vi "line_regulation_test.vi"() -> ()   [LabVIEW 2020, in "line_regulation_test.lvlib"]
uses:
  line_regulation_test.lvlib
  typedefs/test_inputs.ctl
  typedefs/test_results.ctl
  typedefs/instrument_resources.ctl
  <vilib>/addons/_JKI Toolkits/State Machine/_JKI_lib_State_Machine.llb/Select State(s)_err__jki_lib_state_machine.vi
  drivers/Agilent 34401/Public/Data/Read (Single Point).vi
  drivers/Agilent 34401/Agilent 34401.lvlib
  drivers/Agilent E364X Series/Agilent E364X Series.lvlib
  drivers/Agilent 3352X Series/Agilent 3352X Series.lvlib
  drivers/Agilent B2900 Series/Agilent B2900 Series.lvlib
panel:
  in  "UI Tab":enum32{"Test", "Instrument Resources"}(tab)
  in  "test_inputs":T1={"Vin 1 (V)"=36.0, "Iin Limit (A)"=0.1, "ILoad (A)"=0.0, "Vdd (V)"=36.0, "IVdd Limit (A)"=0.1, "Vin 2 (V)"=10.0} {"Vin 2 (V)" format="%#_6p"; "IVdd Limit (A)" format="%#_6p"; "Vdd (V)" format="%#_6p"; "ILoad (A)" format="%#_6p"; "Iin Limit (A)" format="%#_6p"; "Vin 1 (V)" format="%#_6p"}
  out "Output Results":T2
  in  "instrument_resources":T3={"Vin Voltage DMM"="Vin_Volt", "Vin Current DMM"="Vin_Current", "Vout Voltage DMM"="Vout Voltage DMM", "Vout Current DMM"="Vout_Current", "Eload"="Eload", "FSW_Source"="FSW", "Vin_supply"="Vin_supply", "Vdd_supply"="Vin_supply"}
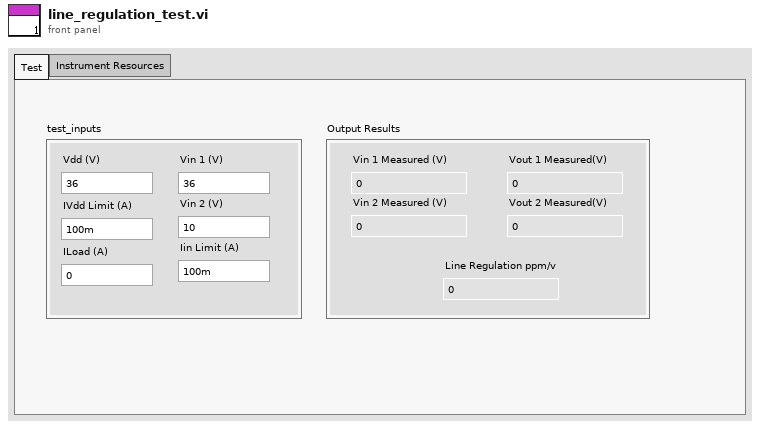
[diagram p1: front panel]
types:
  T1 = typedef "line_regulation_test.lvlib/test_inputs.ctl" = cluster{"Vin 1 (V)":dbl, "Iin Limit (A)":dbl, "ILoad (A)":dbl, "Vdd (V)":dbl, "IVdd Limit (A)":dbl, "Vin 2 (V)":dbl}
  T2 = typedef "line_regulation_test.lvlib/test_results.ctl" = cluster{"Vin 1 Measured (V)":dbl, "Vin 2 Measured (V)":dbl, "Line Regulation ppm/v":dbl, "Vout 1 Measured(V)":dbl, "Vout 2 Measured(V)":dbl}
  T3 = typedef "line_regulation_test.lvlib/instrument_resources.ctl" = cluster{"Vin Voltage DMM":refnum<visa-resource-name>, "Vin Current DMM":refnum<visa-resource-name>, "Vout Voltage DMM":refnum<visa-resource-name>, "Vout Current DMM":refnum<visa-resource-name>, "Eload":refnum<visa-resource-name>, "FSW_Source":refnum<visa-resource-name>, "Vin_supply":refnum<visa-resource-name>, "Vdd_supply":refnum<visa-resource-name>}
  T4 = cluster{"test_inputs":T1, "output_results":T2, "instrument_resources":T3}
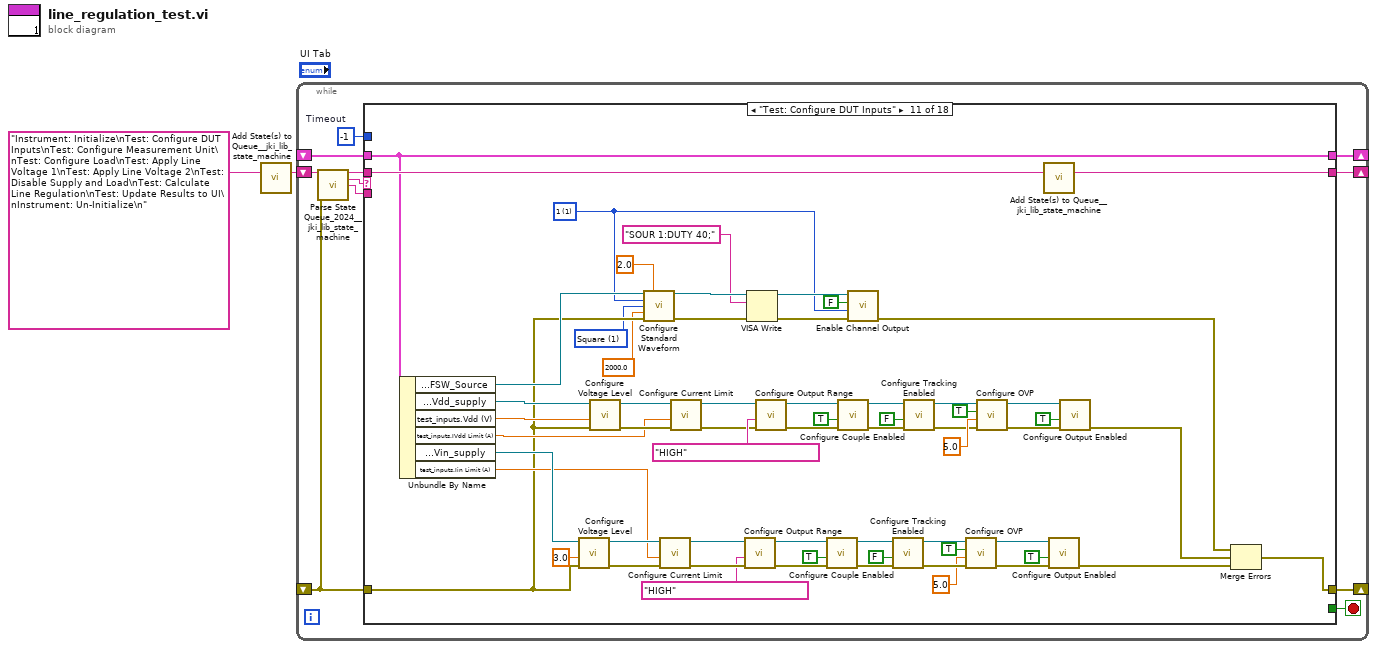
[diagram p0: block diagram]
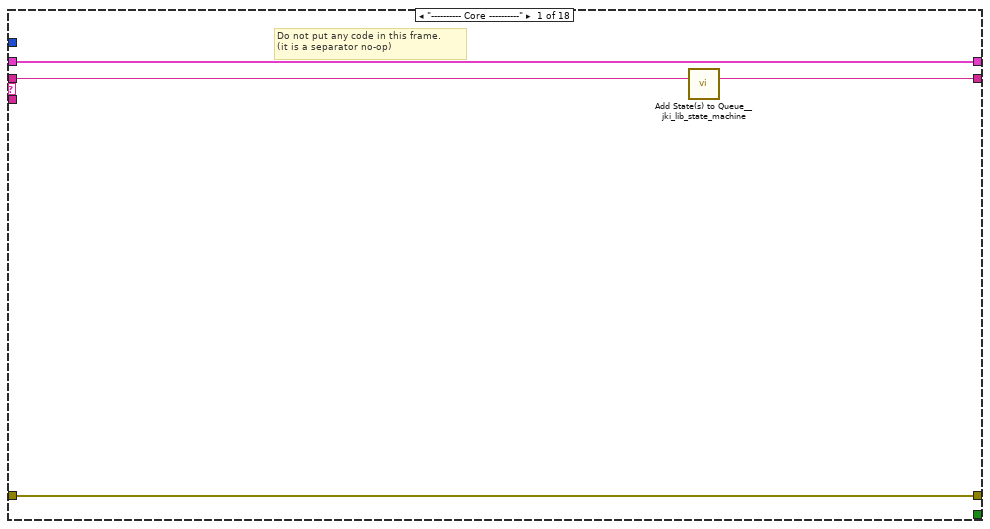
[diagram p2: hidden frame]
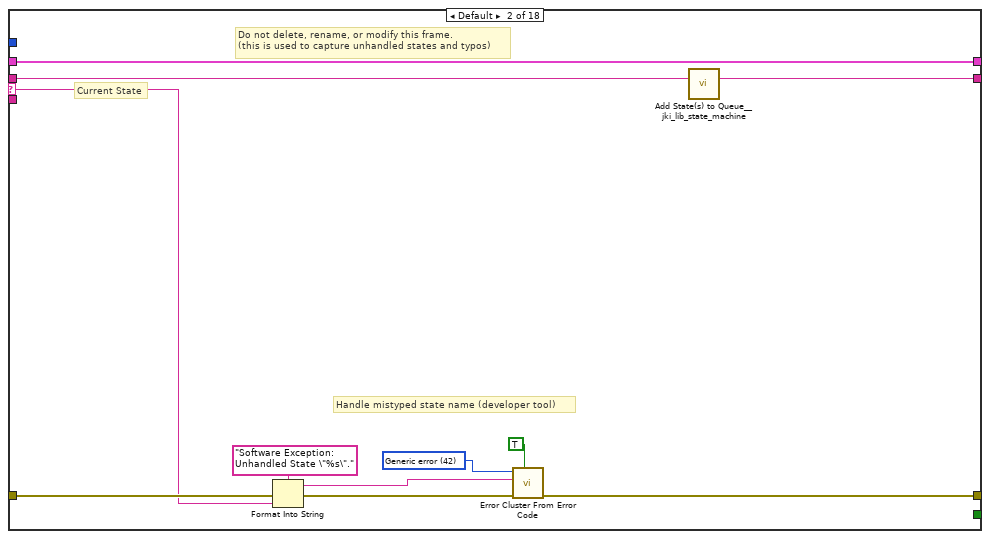
[diagram p3: hidden frame]
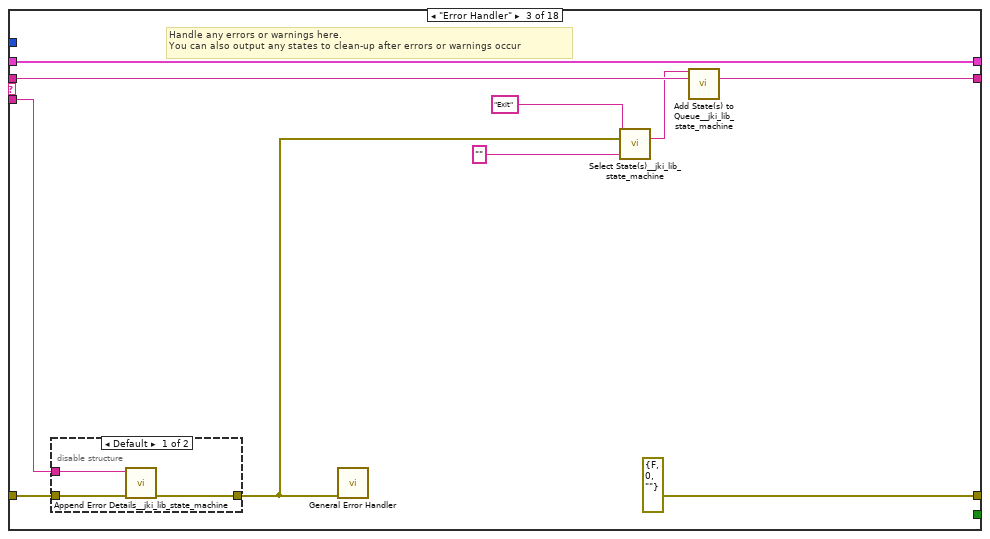
[diagram p4: hidden frame]
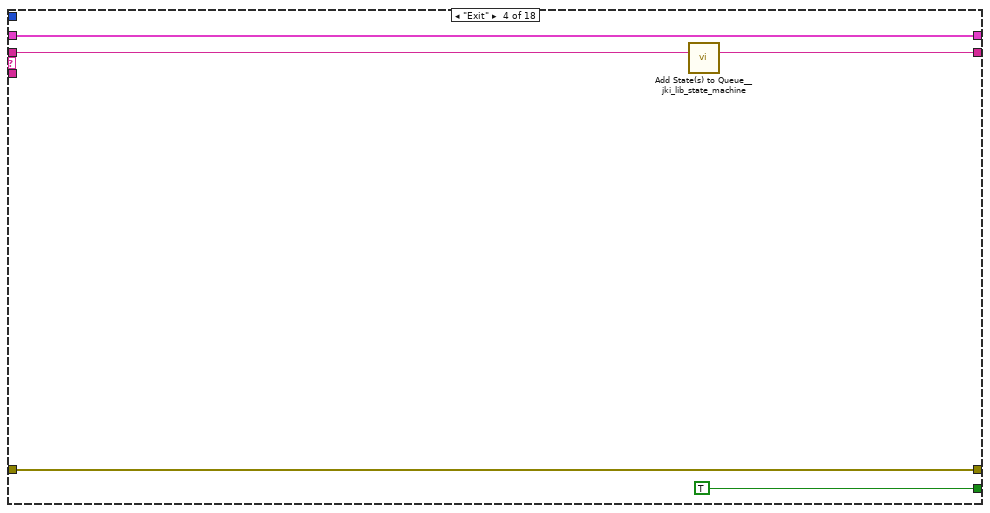
[diagram p6: hidden frame]
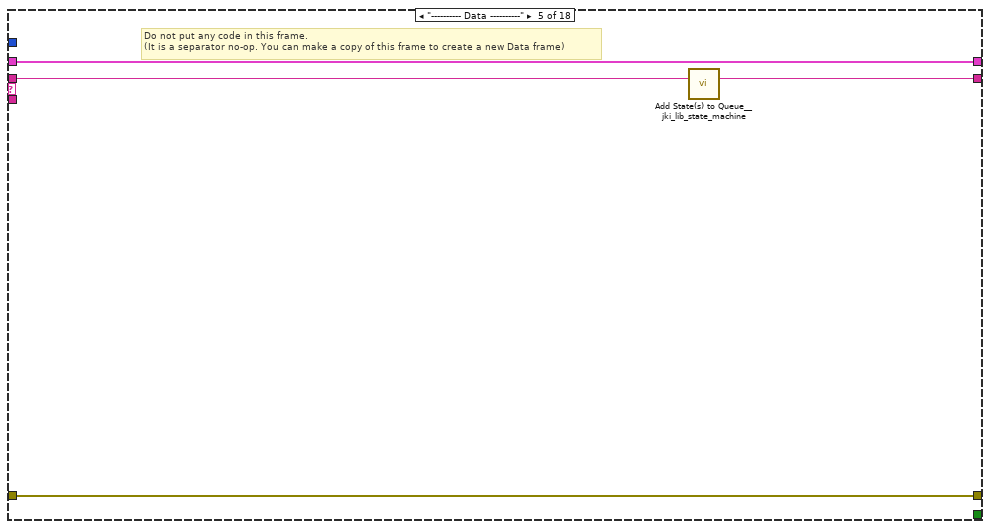
[diagram p7: hidden frame]
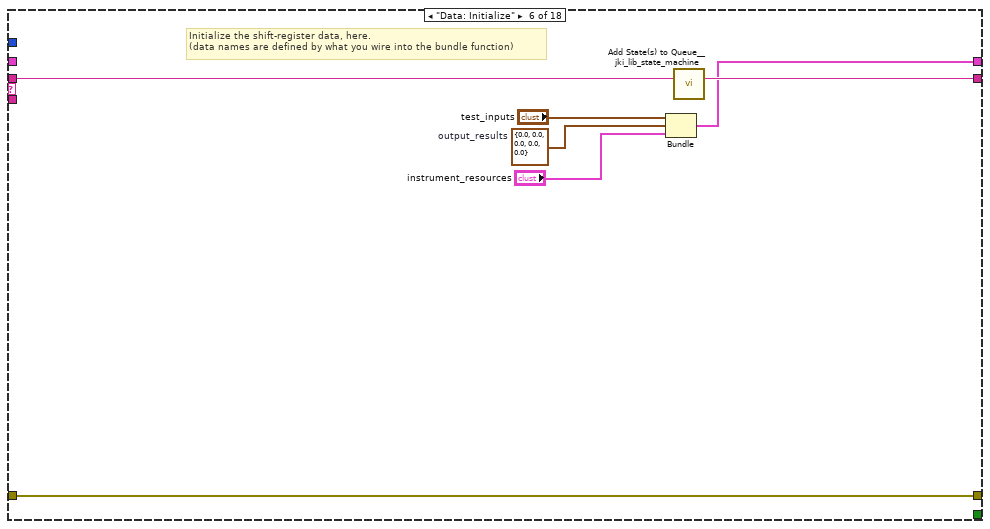
[diagram p8: hidden frame]
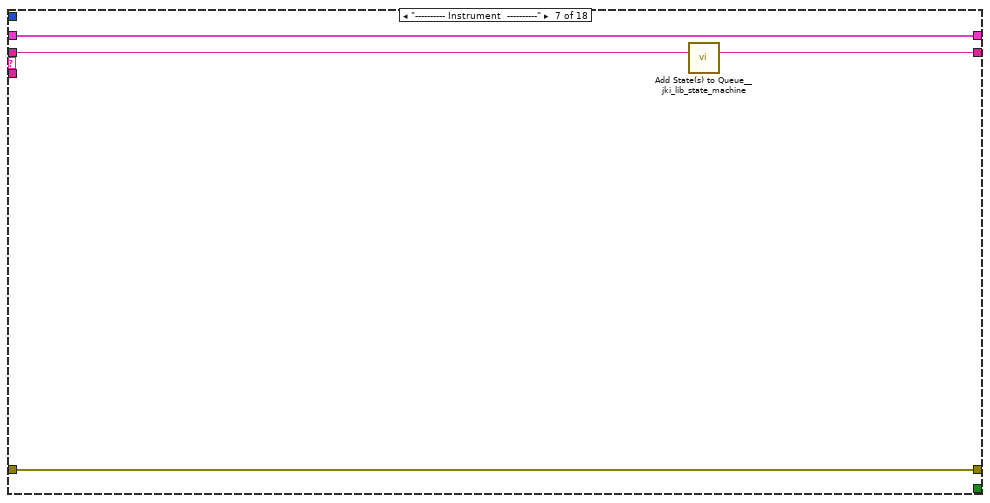
[diagram p9: hidden frame]
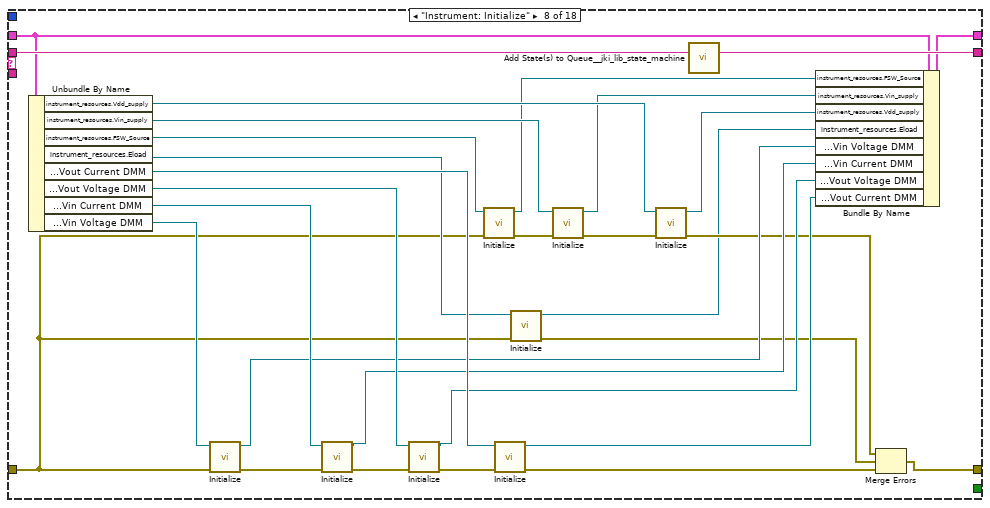
[diagram p10: hidden frame]
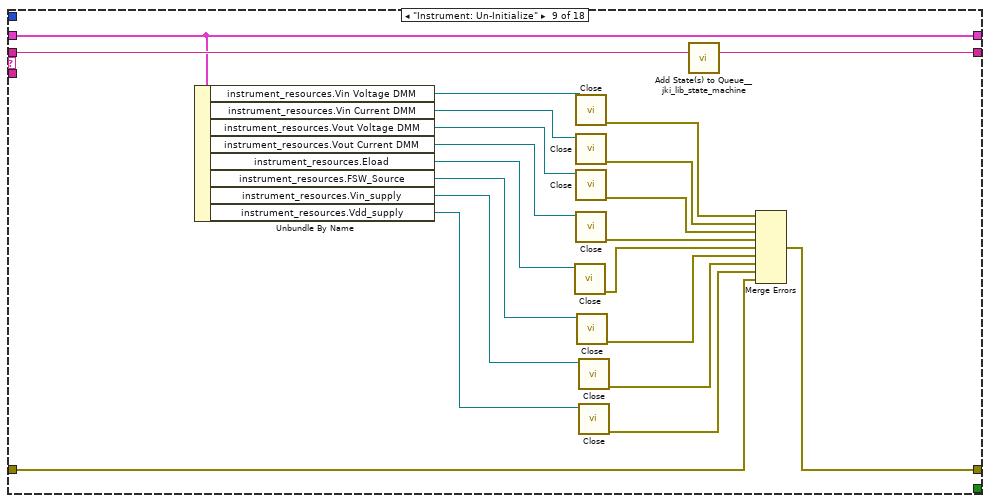
[diagram p11: hidden frame]
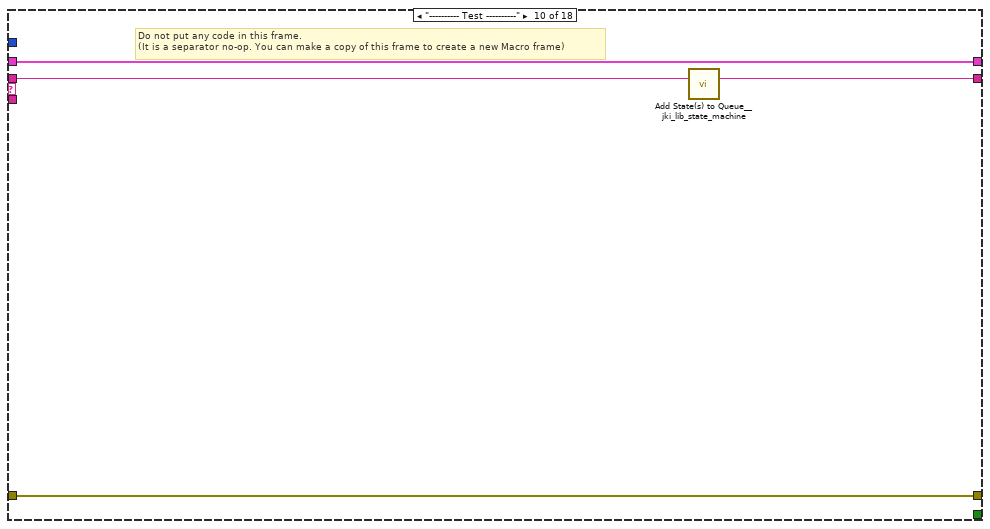
[diagram p12: hidden frame]
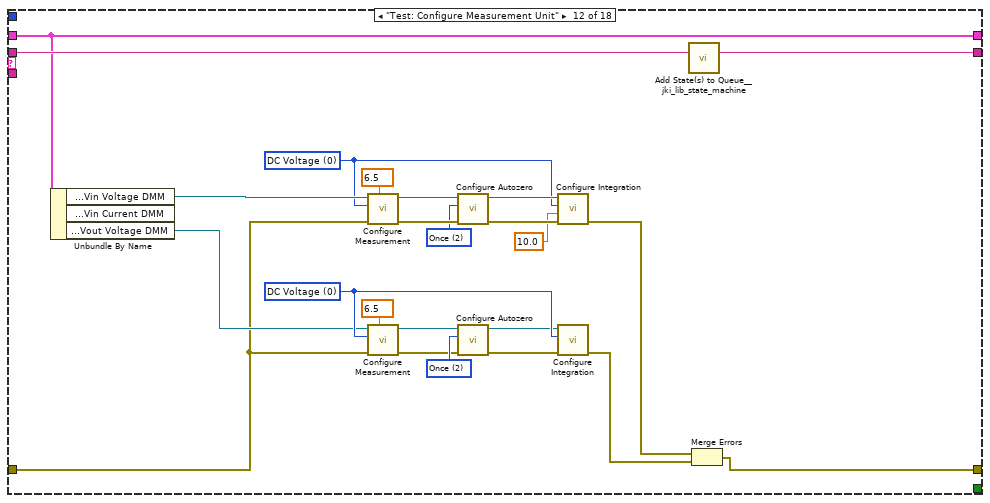
[diagram p13: hidden frame]
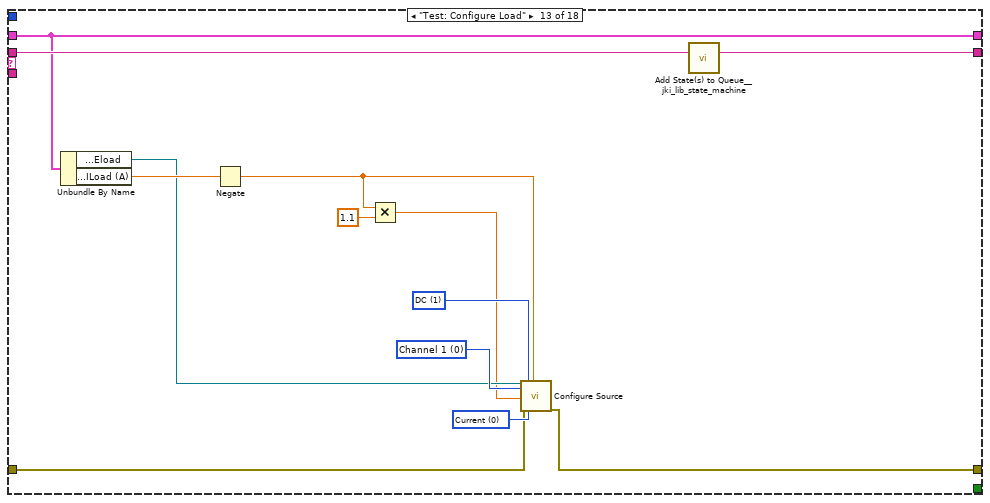
[diagram p14: hidden frame]
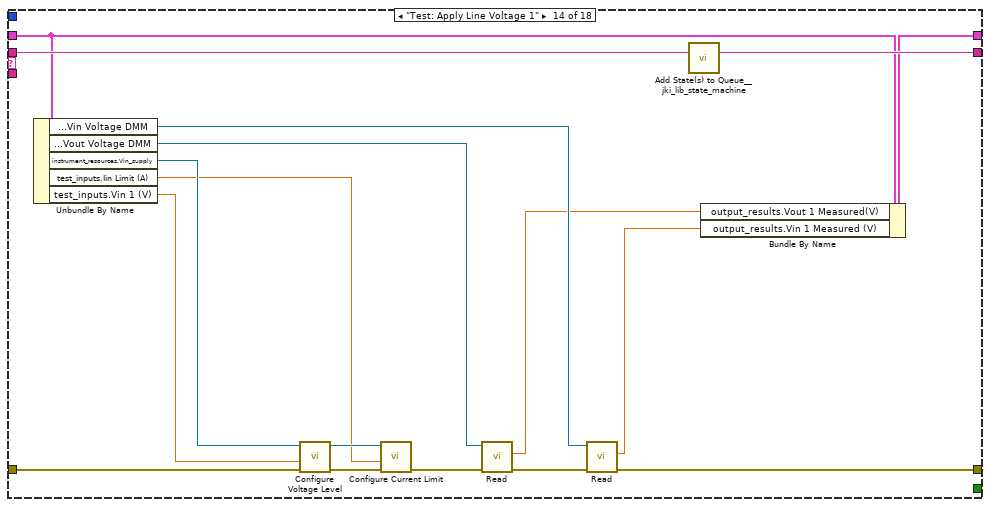
[diagram p15: hidden frame]
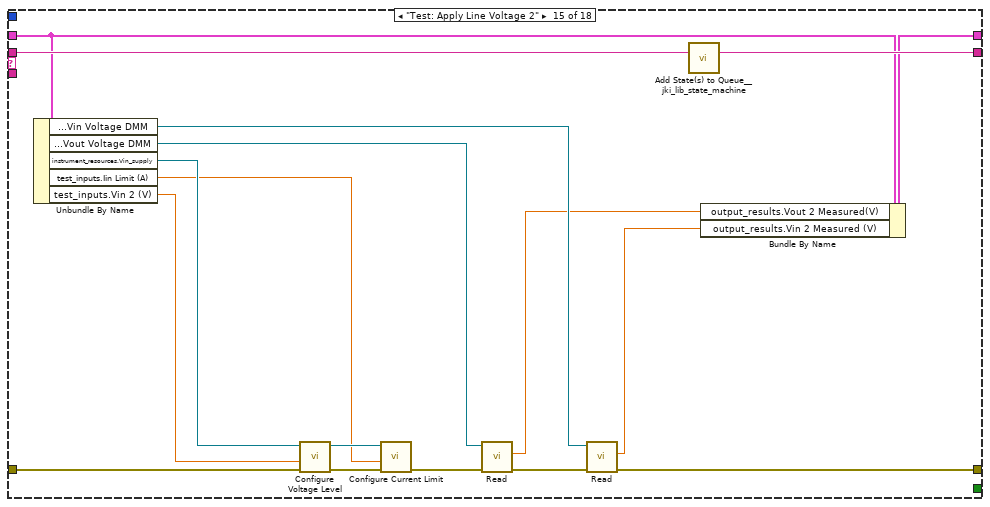
[diagram p16: hidden frame]
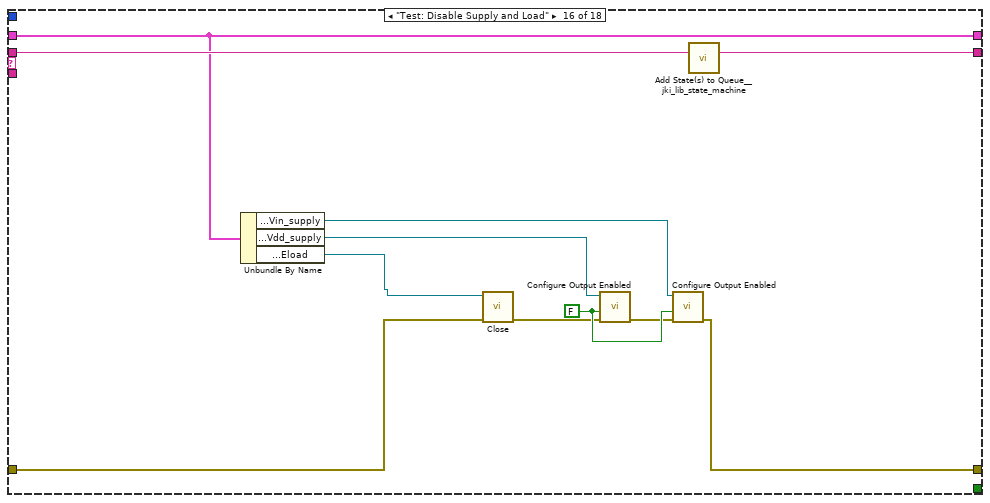
[diagram p17: hidden frame]
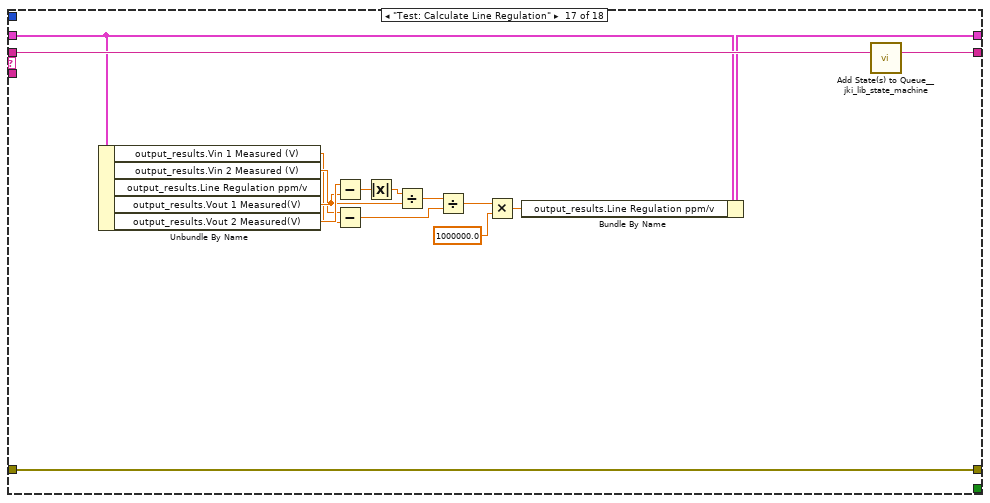
[diagram p18: hidden frame]
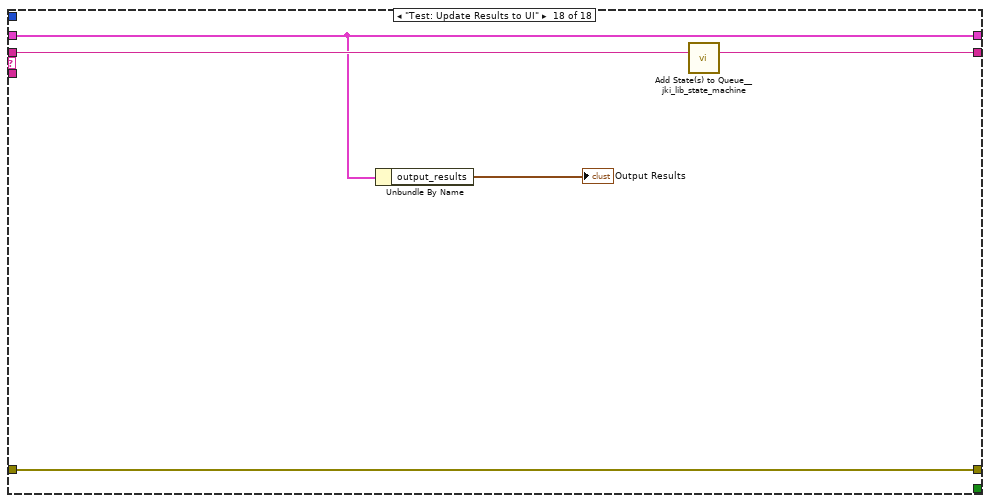
[diagram p19: hidden frame]
diagram:
  n1 = call <vilib>:"Add State(s) to Queue__jki_lib_state_machine.vi"("State(s) in (\"\")"="Instrument: Initialize\nTest: Configure DUT Inputs\nTest: Configure Measurement Unit\nTest: Configure Load\nTest: Apply Line Voltage 1\nTest: Apply Line Voltage 2\nTest: Disable Supply and Load\nTest: Calculate Line Regulation\nTest: Update Results to UI\nInstrument: Un-Initialize\n") -> ("States Out"=w2:string)  [unwired: 14 in]
  n2 = while {
    shift-right: [w6] -> _
    shift-left: _ -> [w5]
    shift-right: [w9] -> _
    shift-left: _ -> [w3]
    shift-right: [w8] -> _
    shift-left: w2 -> [w10]
    stop <- w7 stop-if-true
    w4 = -1  # Timeout
    n3 = call <vilib>:"Parse State Queue_2024__jki_lib_state_machine.vi"("State Queue"=w10, "Error In (no error)"=w3) -> ("Remaining States"=w12:string, "Current State"=w13:string, "Arguments"=w11:string)  [unwired: 11 in]
    n4 = case shown="\"Test: Configure DUT Inputs\"" w13 {
      selector: w13 -> [_ w18 _ _ _ _ _ _ _ _ _ _ _ _ _ _ _ _]
      tunnel: w12 -> [w17 w22 w38 w47 w51 w58 w62 w92 w113 w117 w178 w202 w215 w232 w249 w260 w276 w281]
      tunnel: w11 -> [_ _ w33 _ _ _ _ _ _ _ _ _ _ _ _ _ _ _]
      tunnel: w5 -> [w14 w20 w35 w45 w48 _ w59 w70 w111 w114 w176 w200 w213 w219 w236 w258 w272 w278]
      tunnel: [w15 w24 errorcluster {"status"=FALSE, "code"=0, "source"=""} ("error out") w44 w49 w55 w60 w67 w96 w115 w124 w180 w206 w217 w234 w253 w274 w279] -> w9
      tunnel: w3 -> [w15 w23 w34 w44 w49 w55 w60 w64 w95 w115 w133 w182 w207 w228 w245 w252 w274 w279]
      tunnel: [w16 w21 w37 w46 w50 w57 w61 w91 w112 w116 w177 w201 w214 w231 w248 w259 w275 w280] -> w8
      tunnel: [_ _ _ TRUE _ _ _ _ _ _ _ _ _ _ _ _ _ _] -> w7
      tunnel: [w14 w20 w35 w45 w48 w56 w59 w71 w111 w114 w176 w200 w213 w220 w237 w258 w273 w278] -> w6
      tunnel: w4 -> [_ _ _ _ _ _ _ _ _ _ _ _ _ _ _ _ _ _]
      frame "---------- Core ----------" {
        # "Do not put any code in this frame.\n(it is a separator no-op)"
        n5 = call <vilib>:"Add State(s) to Queue__jki_lib_state_machine.vi"("State(s) in (\"\")"=w17) -> ("States Out"=w16:string)  [unwired: 14 in]
      }
      frame Default {
        w27 = 42 items=["No error", "Argument error", "Memory is full", "Out of zone", "End of file", "File already open", "Generic file I/O error", "File not found", "File permission error", "Disk is full", "Duplicate path", "Too many files open", "System feature not enabled", "Resource file not found", "Cannot add resource", "Resource not found", "Image not found", "Image memory error", "Pen does not exist", "Config type invalid", "Config token not found", "Config parse error", "Config memory error", "Bad external code format", "Bad external code offset", "External code not present", "Null window", "Destroy window error", "Null menu", "Print aborted", "Bad print record", "Print driver error", "Windows error during printing", "Memory error during printing", "Print dialog error", "Generic print error", "Invalid device refnum", "Device not found", "Device parameter error", "Device unit error", "Cannot open device", "Device call aborted", "Generic error", "Cancelled by user", "Object ID too low", "Object ID too high", "Object not in heap", "Unknown heap", "Unknown object (invalid DefProc)", "Unknown object (DefProc not in table)", "Message out of range", "Invalid (null) method", "Unknown message", "Manager call not supported", "Bad address", "Network operation in progress", "Network operation timed out", "Connection is busy", "Network attribute not supported", "Network error", "Address in use", "System out of memory", "Connection aborted", "Connection refused", "Not connected", "Already connected", "Connection closed", "Initialization error (interapplication manager)", "Bad occurrence", "Wait on unbound occurrence handler", "Occurrence queue overflow", "Datalog type conflict", "Unused", "Unrecognized type (interapplication manager)", "Memory corrupt", "Failed to make temporary DLL", "Old CIN version", "Drag socket not found", "Failed to load drop-object", "Failed to register OLE object", "Failed to release OLE object", "Format specifier type mismatch", "Unknown format specifier", "Too few format specifiers", "Too many format specifiers", "Scan failed", "Newer CIN version", "Error converting to variant", "Runtime menu error", "Password tampered", "Variant attribute not found", "Incompatible variant data type", "Event data is not available", "Event Store is not present", "Occurrence is not found", "Event Queue is not created", "Event info is not available", "Refnum passed is NULL", "Error retrieving Class GUID", "Error retrieving CoClass GUID", "Error retrieving TypeLib GUID.", "Bad built application magic bytes.", "Specific driver is different from the specific driver associated with the Logical Name.", "There is no session opened to the class driver.", "Max Error", "MAX - Error with config objects", "MAX - Error loading configuration", "MAX - Group not supported"]
        # "Current State"
        # "Do not delete, rename, or modify this frame.\n(this is used to capture unhandled states and typos)"
        # "Handle mistyped state name (developer tool)"
        n6 = Format Into String(format string="Software Exception: Unhandled State \"%s\"." ("message"), error in=w23, w18) -> (resulting string=w26:string, error out=w25:errorcluster)  [unwired: 1 in]
        n7 = call <vilib>:"Error Cluster From Error Code.vi"("show call chain? (False)"=TRUE, "error in (no error)"=w25, "error message (\"\")"=w26, "error code (0)"=w27) -> ("error out"=w24:errorcluster)  [unwired: 5 in]
        n8 = call <vilib>:"Add State(s) to Queue__jki_lib_state_machine.vi"("State(s) in (\"\")"=w22) -> ("States Out"=w21:string)  [unwired: 14 in]
      }
      frame "Error Handler" {
        # "Handle any errors or warnings here.\nYou can also output any states to clean-up after errors or warnings occur"
        n9 = disable-structure shown="Default" {
          disable-tunnel: w34 -> [w41 w42]
          disable-tunnel: w33 -> [w40 _]
          disable-tunnel: [w39 w42] -> w32
          frame condition #0 (active) {
            n10 = call <vilib>:"Append Error Details__jki_lib_state_machine.vi"("error in (no error)"=w41, "Previous State and Argument(s)"=w40) -> ("error out"=w39:errorcluster)  [unwired: 9 in]
          }
          frame condition #1 {
          }
        }
        n11 = call <vilib>:"General Error Handler.vi"("error in (no error)"=w32) -> ()  [unwired: 10 in, 5 out]
        n12 = call-poly <vilib>:"Select State(s)__jki_lib_state_machine.vi"("State(s) if True (\"\")"="Exit", "Select"=w32, "State(s) if False (\"\")"="") -> ("States Out"=w30:string)  [unwired: 12 in]
        n13 = call <vilib>:"Add State(s) to Queue__jki_lib_state_machine.vi"("State(s) in Front (\"\")"=w30, "State(s) in (\"\")"=w38) -> ("States Out"=w37:string)  [unwired: 13 in]
      }
      frame "Exit" {
        n14 = call <vilib>:"Add State(s) to Queue__jki_lib_state_machine.vi"("State(s) in (\"\")"=w47) -> ("States Out"=w46:string)  [unwired: 14 in]
      }
      frame "---------- Data ----------" {
        # "Do not put any code in this frame.\n(It is a separator no-op. You can make a copy of this frame to create a new Data frame)"
        n15 = call <vilib>:"Add State(s) to Queue__jki_lib_state_machine.vi"("State(s) in (\"\")"=w51) -> ("States Out"=w50:string)  [unwired: 14 in]
      }
      frame "Data: Initialize" {
        w53 = T2 {"Vin 1 Measured (V)"=0.0, "Vin 2 Measured (V)"=0.0, "Line Regulation ppm/v"=0.0, "Vout 1 Measured(V)"=0.0, "Vout 2 Measured(V)"=0.0}  # output_results
        # "Initialize the shift-register data, here.\n(data names are defined by what you wire into the bundle function)"
        n16 = Bundle("test_inputs"="test_inputs", "output_results"=w53, "instrument_resources"="instrument_resources") -> (w56:T4)  [unwired: 1 in]
        n17 = call <vilib>:"Add State(s) to Queue__jki_lib_state_machine.vi"("State(s) in (\"\")"=w58) -> ("States Out"=w57:string)  [unwired: 14 in]
      }
      frame "---------- Instrument  ----------" {
        n18 = call <vilib>:"Add State(s) to Queue__jki_lib_state_machine.vi"("State(s) in (\"\")"=w62) -> ("States Out"=w61:string)  [unwired: 14 in]
      }
      frame "Instrument: Initialize" {
        n19 = Unbundle By Name(w70) -> ("instrument_resources.Vdd_supply"=w83:refnum<visa-resource-name>, "instrument_resources.Vin_supply"=w84:refnum<visa-resource-name>, "instrument_resources.FSW_Source"=w85:refnum<visa-resource-name>, "instrument_resources.Eload"=w66:refnum<visa-resource-name>, "instrument_resources.Vout Current DMM"=w79:refnum<visa-resource-name>, "instrument_resources.Vout Voltage DMM"=w80:refnum<visa-resource-name>, "instrument_resources.Vin Current DMM"=w81:refnum<visa-resource-name>, "instrument_resources.Vin Voltage DMM"=w82:refnum<visa-resource-name>)
        n20 = call "Initialize.vi"("error in (no error)"=w64, "VISA resource name"=w82) -> ("error out"=w88:errorcluster, "VISA resource name out"=w75:refnum<visa-resource-name>)  [unwired: 8 in]
        n21 = call "Initialize.vi"("error in (no error)"=w88, "VISA resource name"=w81) -> ("error out"=w90:errorcluster, "VISA resource name out"=w74:refnum<visa-resource-name>)  [unwired: 8 in]
        n22 = call "Initialize.vi"("error in (no error)"=w90, "VISA resource name"=w80) -> ("error out"=w89:errorcluster, "VISA resource name out"=w73:refnum<visa-resource-name>)  [unwired: 8 in]
        n23 = call "Initialize.vi"("error in (no error)"=w64, "VISA resource name"=w85) -> ("error out"=w87:errorcluster, "VISA resource name out"=w78:refnum<visa-resource-name>)  [unwired: 8 in]
        n24 = call "Initialize.vi"("error in (no error)"=w89, "VISA resource name"=w79) -> ("error out"=w68:errorcluster, "VISA resource name out"=w72:refnum<visa-resource-name>)  [unwired: 8 in]
        n25 = call "Initialize.vi"("error in (no error)"=w64, "VISA resource name"=w66) -> ("error out"=w63:errorcluster, "VISA resource name out"=w65:refnum<visa-resource-name>)  [unwired: 8 in]
        n26 = call "Initialize.vi"("error in (no error)"=w87, "VISA resource name"=w84) -> ("error out"=w86:errorcluster, "VISA resource name out"=w77:refnum<visa-resource-name>)  [unwired: 8 in]
        n27 = call "Initialize.vi"("error in (no error)"=w86, "VISA resource name"=w83) -> ("error out"=w69:errorcluster, "VISA resource name out"=w76:refnum<visa-resource-name>)  [unwired: 8 in]
        n28 = call <vilib>:"Add State(s) to Queue__jki_lib_state_machine.vi"("State(s) in (\"\")"=w92) -> ("States Out"=w91:string)  [unwired: 14 in]
        n29 = Bundle By Name(cluster=w70, "instrument_resources.FSW_Source"=w78, "instrument_resources.Vin_supply"=w77, "instrument_resources.Vdd_supply"=w76, "instrument_resources.Eload"=w65, "instrument_resources.Vin Voltage DMM"=w75, "instrument_resources.Vin Current DMM"=w74, "instrument_resources.Vout Voltage DMM"=w73, "instrument_resources.Vout Current DMM"=w72) -> (w71:T4)
        n30 = Merge Errors(w69, w63, w68) -> (w67:errorcluster)
      }
      frame "Instrument: Un-Initialize" {
        n31 = Unbundle By Name(w111) -> ("instrument_resources.Vin Voltage DMM"=w110:refnum<visa-resource-name>, "instrument_resources.Vin Current DMM"=w109:refnum<visa-resource-name>, "instrument_resources.Vout Voltage DMM"=w108:refnum<visa-resource-name>, "instrument_resources.Vout Current DMM"=w107:refnum<visa-resource-name>, "instrument_resources.Eload"=w94:refnum<visa-resource-name>, "instrument_resources.FSW_Source"=w106:refnum<visa-resource-name>, "instrument_resources.Vin_supply"=w105:refnum<visa-resource-name>, "instrument_resources.Vdd_supply"=w104:refnum<visa-resource-name>)
        n32 = call "Close.vi"("VISA resource name"=w94) -> ("error out"=w93:errorcluster)  [unwired: 10 in]
        n33 = call "Close.vi"("VISA resource name"=w110) -> ("error out"=w103:errorcluster)  [unwired: 10 in]
        n34 = call "Close.vi"("VISA resource name"=w109) -> ("error out"=w102:errorcluster)  [unwired: 10 in]
        n35 = call "Close.vi"("VISA resource name"=w108) -> ("error out"=w101:errorcluster)  [unwired: 10 in]
        n36 = call "Close.vi"("VISA resource name"=w107) -> ("error out"=w100:errorcluster)  [unwired: 10 in]
        n37 = call "Close.vi"("VISA resource name"=w106) -> ("error out"=w99:errorcluster)  [unwired: 10 in]
        n38 = call "Close.vi"("VISA resource name"=w105) -> ("error out"=w98:errorcluster)  [unwired: 10 in]
        n39 = call "Close.vi"("VISA resource name"=w104) -> ("error out"=w97:errorcluster)  [unwired: 10 in]
        n40 = call <vilib>:"Add State(s) to Queue__jki_lib_state_machine.vi"("State(s) in (\"\")"=w113) -> ("States Out"=w112:string)  [unwired: 14 in]
        n41 = Merge Errors(w103, w102, w101, w100, w93, w99, w98, w97, w95) -> (w96:errorcluster)
      }
      frame "---------- Test ----------" {
        # "Do not put any code in this frame.\n(It is a separator no-op. You can make a copy of this frame to create a new Macro frame)"
        n42 = call <vilib>:"Add State(s) to Queue__jki_lib_state_machine.vi"("State(s) in (\"\")"=w117) -> ("States Out"=w116:string)  [unwired: 14 in]
      }
      frame "Test: Configure DUT Inputs" {
        w122 = 1 items=["Sine"=0, "Square"=1, "Ramp"=2, "Noise"=3, "DC"=4, "Triangle"=5, "Pulse"=6, "Sinc"=11, "D-Lorentz"=12, "Gaussian"=13, "Expo Fall"=14, "Expo Rise"=15, "Haversine"=16] ("Waveform Function (0: Sine)")
        w120 = 1 items=["1"=1, "2"=2] ("Channel (1: 1)")
        n43 = Unbundle By Name(w176) -> ("instrument_resources.FSW_Source"=w134:refnum<visa-resource-name>, "instrument_resources.Vdd_supply"=w137:refnum<visa-resource-name>, "test_inputs.Vdd (V)"=w136:dbl, "test_inputs.IVdd Limit (A)"=w135:dbl, "instrument_resources.Vin_supply"=w175:refnum<visa-resource-name>, "test_inputs.Iin Limit (A)"=w156:dbl)
        n44 = call "Configure Voltage Level.vi"("error in (no error)"=w133, "Level (0.0 Volts)"=3.0, "VISA resource name"=w175) -> ("error out"=w174:errorcluster, "VISA resource name out"=w170:refnum<visa-resource-name>)  [unwired: 7 in]
        n45 = call "Configure Voltage Level.vi"("error in (no error)"=w133, "Level (0.0 Volts)"=w136, "VISA resource name"=w137) -> ("error out"=w138:errorcluster, "VISA resource name out"=w142:refnum<visa-resource-name>)  [unwired: 7 in]
        n46 = call "Configure Standard Waveform.vi"("VISA resource name"=w134, "Amplitude (0.1 Vpp)"=2.0, "Channel (1: 1)"=w120, "Waveform Function (0: Sine)"=w122, "Frequency/Sample Rate/Bandwidth (1000 Hz)"=2000.0, "error in (no error)"=w133) -> ("VISA resource name out"=w130:refnum<visa-resource-name>, "error out"=w132:errorcluster)  [unwired: 8 in]
        n47 = call "Configure Current Limit.vi"("error in (no error)"=w174, "Current Limit (0.0 Amps)"=w156, "VISA resource name"=w170) -> ("error out"=w173:errorcluster, "VISA resource name out"=w169:refnum<visa-resource-name>)  [unwired: 7 in]
        n48 = call "Configure Current Limit.vi"("error in (no error)"=w138, "Current Limit (0.0 Amps)"=w135, "VISA resource name"=w142) -> ("error out"=w139:errorcluster, "VISA resource name out"=w143:refnum<visa-resource-name>)  [unwired: 7 in]
        n49 = call "Configure Output Range.vi"("error in (no error)"=w173, "Range (High Voltage / Low Current)"="HIGH", "VISA resource name"=w169) -> ("error out"=w172:errorcluster, "VISA resource name out"=w168:refnum<visa-resource-name>)  [unwired: 7 in]
        n50 = VISA Write(VISA resource name=w130, write buffer="SOUR 1:DUTY 40;", error in (no error)=w132) -> (VISA resource name out=w129:refnum<visa-resource-name>, error out=w131:errorcluster)  [unwired: 1 out]
        n51 = call "Configure Output Range.vi"("error in (no error)"=w139, "Range (High Voltage / Low Current)"="HIGH", "VISA resource name"=w143) -> ("error out"=w140:errorcluster, "VISA resource name out"=w144:refnum<visa-resource-name>)  [unwired: 7 in]
        n52 = call "Configure Couple Enabled.vi"("error in (no error)"=w172, "Coupling Enabled (F: Off)"=TRUE, "VISA resource name"=w168) -> ("error out"=w171:errorcluster, "VISA resource name out"=w167:refnum<visa-resource-name>)  [unwired: 7 in]
        n53 = call "Configure Couple Enabled.vi"("error in (no error)"=w140, "Coupling Enabled (F: Off)"=TRUE, "VISA resource name"=w144) -> ("error out"=w141:errorcluster, "VISA resource name out"=w145:refnum<visa-resource-name>)  [unwired: 7 in]
        n54 = call "Enable Channel Output.vi"("error in (no error)"=w131, "Channel (1: 1)"=w120, "Enable Output (T: Enable)"=FALSE ("Enable Output  (T: Enable)"), "VISA resource name"=w129) -> ("error out"=w125:errorcluster)  [unwired: 6 in, 1 out]
        n55 = call "Configure Tracking Enabled.vi"("error in (no error)"=w171, "Tracking Enabled (F: Off)"=FALSE, "VISA resource name"=w167) -> ("error out"=w163:errorcluster, "VISA resource name out"=w161:refnum<visa-resource-name>)  [unwired: 7 in]
        n56 = call "Configure Tracking Enabled.vi"("error in (no error)"=w141, "Tracking Enabled (F: Off)"=FALSE, "VISA resource name"=w145) -> ("error out"=w149:errorcluster, "VISA resource name out"=w151:refnum<visa-resource-name>)  [unwired: 7 in]
        n57 = call "Configure OVP.vi"("error in (no error)"=w163, "Limit (22.0 Volts)"=5.0, "OVP Enabled (T: On)"=TRUE, "VISA resource name"=w161) -> ("error out"=w159:errorcluster, "VISA resource name out"=w158:refnum<visa-resource-name>)  [unwired: 6 in]
        n58 = call "Configure OVP.vi"("error in (no error)"=w149, "Limit (22.0 Volts)"=5.0, "OVP Enabled (T: On)"=TRUE, "VISA resource name"=w151) -> ("error out"=w153:errorcluster, "VISA resource name out"=w154:refnum<visa-resource-name>)  [unwired: 6 in]
        n59 = call <vilib>:"Add State(s) to Queue__jki_lib_state_machine.vi"("State(s) in (\"\")"=w178) -> ("States Out"=w177:string)  [unwired: 14 in]
        n60 = call "Configure Output Enabled.vi"("error in (no error)"=w159, "Output Enabled (F: Off)"=TRUE, "VISA resource name"=w158) -> ("error out"=w127:errorcluster)  [unwired: 7 in, 1 out]
        n61 = call "Configure Output Enabled.vi"("error in (no error)"=w153, "Output Enabled (F: Off)"=TRUE, "VISA resource name"=w154) -> ("error out"=w126:errorcluster)  [unwired: 7 in, 1 out]
        n62 = Merge Errors(w125, w126, w127) -> (w124:errorcluster)
      }
      frame "Test: Configure Measurement Unit" {
        w190 = 6.5 items=["4.5"=4.5, "5.5"=5.5, "6.5"=6.5] ("Manual Resolution (5.5 Digits)")
        w189 = u16 2 items=["On", "Off", "Once"] ("Autozero  (0: On)")
        w188 = u16 0 items=["DC Voltage", "AC Voltage", "2 - Wire Resistance", "4 - Wire Resistance", "DC Current", "AC Current", "Frequency", "Period", "Continuity", "Diode Checking", "VDC:VDC Ratio", "Temperature", "Capacitance"] ("Function (0: DC Voltage)")
        w191 = 6.5 items=["4.5"=4.5, "5.5"=5.5, "6.5"=6.5] ("Manual Resolution (5.5 Digits)")
        w192 = u16 2 items=["On", "Off", "Once"] ("Autozero  (0: On)")
        w193 = 10.0 items=["0.001"=0.001, "0.002"=0.002, "0.006"=0.006, "0.02"=0.02, "0.06"=0.06, "0.2"=0.2, "1"=1.0, "10"=10.0, "100"=100.0] ("Integration Time (1 PLCs)")
        w194 = u16 0 items=["DC Voltage", "AC Voltage", "2 - Wire Resistance", "4 - Wire Resistance", "DC Current", "AC Current", "Frequency", "Period", "Continuity", "Diode Checking", "VDC:VDC Ratio", "Temperature", "Capacitance"] ("Function (0: DC Voltage)")
        n63 = Unbundle By Name(w200) -> ("instrument_resources.Vin Voltage DMM"=w199:refnum<visa-resource-name>, "instrument_resources.Vout Voltage DMM"=w183:refnum<visa-resource-name>)  [unwired: 1 out]
        n64 = call "Configure Measurement.vi"("Manual Resolution (5.5 Digits)"=w191, "error in (no error)"=w182, "Function (0: DC Voltage)"=w194, "VISA resource name"=w199) -> ("error out"=w197:errorcluster, "VISA resource name out"=w198:refnum<visa-resource-name>)  [unwired: 6 in]
        n65 = call "Configure Measurement.vi"("Manual Resolution (5.5 Digits)"=w190, "error in (no error)"=w182, "Function (0: DC Voltage)"=w188, "VISA resource name"=w183) -> ("error out"=w185:errorcluster, "VISA resource name out"=w184:refnum<visa-resource-name>)  [unwired: 6 in]
        n66 = call "Configure Autozero.vi"("error in (no error)"=w197, "Autozero  (0: On)"=w192, "VISA resource name"=w198) -> ("error out"=w196:errorcluster, "VISA resource name out"=w195:refnum<visa-resource-name>)  [unwired: 7 in]
        n67 = call "Configure Autozero.vi"("error in (no error)"=w185, "Autozero  (0: On)"=w189, "VISA resource name"=w184) -> ("error out"=w186:errorcluster, "VISA resource name out"=w187:refnum<visa-resource-name>)  [unwired: 7 in]
        n68 = call "Configure Integration.vi"("error in (no error)"=w196, "Integration Time (1 PLCs)"=w193, "Function (0: DC Voltage)"=w194, "VISA resource name"=w195) -> ("error out"=w179:errorcluster)  [unwired: 6 in, 1 out]
        n69 = call "Configure Integration.vi"("error in (no error)"=w186, "Function (0: DC Voltage)"=w188, "VISA resource name"=w187) -> ("error out"=w181:errorcluster)  [unwired: 7 in, 1 out]
        n70 = call <vilib>:"Add State(s) to Queue__jki_lib_state_machine.vi"("State(s) in (\"\")"=w202) -> ("States Out"=w201:string)  [unwired: 14 in]
        n71 = Merge Errors(w179, w181) -> (w180:errorcluster)
      }
      frame "Test: Configure Load" {
        w208 = 0 items=["Current", "Voltage"] ("Source Mode (1: Voltage)")
        w209 = 1 items=["Pulse", "DC"] ("Source Shape (1: DC)")
        w210 = 0 items=["Channel 1", "Channel 2"] ("Channel (0: Channel 1)")
        n72 = Unbundle By Name(w213) -> ("instrument_resources.Eload"=w205:refnum<visa-resource-name>, "test_inputs.ILoad (A)"=w212:dbl)
        n73 = Negate(x=w212) -> (-x=w204:dbl)
        n74 = Multiply(x=w204, y=1.1) -> (x*y=w203:dbl)
        n75 = call "Configure Source.vi"("VISA resource name"=w205, "Channel (0: Channel 1)"=w210, "Source Range (2)"=w203, "error in (no error)"=w207, "Source Shape (1: DC)"=w209, "Source Mode (1: Voltage)"=w208, "Output Level (0)"=w204) -> ("error out"=w206:errorcluster)  [unwired: 11 in, 1 out]
        n76 = call <vilib>:"Add State(s) to Queue__jki_lib_state_machine.vi"("State(s) in (\"\")"=w215) -> ("States Out"=w214:string)  [unwired: 14 in]
      }
      frame "Test: Apply Line Voltage 1" {
        n77 = Unbundle By Name(w219) -> ("instrument_resources.Vin Voltage DMM"=w221:refnum<visa-resource-name>, "instrument_resources.Vout Voltage DMM"=w223:refnum<visa-resource-name>, "instrument_resources.Vin_supply"=w227:refnum<visa-resource-name>, "test_inputs.Iin Limit (A)"=w225:dbl, "test_inputs.Vin 1 (V)"=w226:dbl)
        n78 = call "Configure Voltage Level.vi"("error in (no error)"=w228, "Level (0.0 Volts)"=w226, "VISA resource name"=w227) -> ("error out"=w229:errorcluster, "VISA resource name out"=w230:refnum<visa-resource-name>)  [unwired: 7 in]
        n79 = call "Configure Current Limit.vi"("error in (no error)"=w229, "Current Limit (0.0 Amps)"=w225, "VISA resource name"=w230) -> ("error out"=w224:errorcluster)  [unwired: 7 in, 1 out]
        n80 = call-poly "Read.vi"("error in (no error)"=w224, "VISA resource name"=w223) -> ("error out"=w222:errorcluster, "Measurement"=w218:dbl)  [unwired: 7 in, 1 out]
        n81 = call-poly "Read.vi"("error in (no error)"=w222, "VISA resource name"=w221) -> ("error out"=w217:errorcluster, "Measurement"=w216:dbl)  [unwired: 7 in, 1 out]
        n82 = call <vilib>:"Add State(s) to Queue__jki_lib_state_machine.vi"("State(s) in (\"\")"=w232) -> ("States Out"=w231:string)  [unwired: 14 in]
        n83 = Bundle By Name(cluster=w219, "output_results.Vout 1 Measured(V)"=w218, "output_results.Vin 1 Measured (V)"=w216) -> (w220:T4)
      }
      frame "Test: Apply Line Voltage 2" {
        n84 = Unbundle By Name(w236) -> ("instrument_resources.Vin Voltage DMM"=w238:refnum<visa-resource-name>, "instrument_resources.Vout Voltage DMM"=w240:refnum<visa-resource-name>, "instrument_resources.Vin_supply"=w244:refnum<visa-resource-name>, "test_inputs.Iin Limit (A)"=w242:dbl, "test_inputs.Vin 2 (V)"=w243:dbl)
        n85 = call "Configure Voltage Level.vi"("error in (no error)"=w245, "Level (0.0 Volts)"=w243, "VISA resource name"=w244) -> ("error out"=w246:errorcluster, "VISA resource name out"=w247:refnum<visa-resource-name>)  [unwired: 7 in]
        n86 = call "Configure Current Limit.vi"("error in (no error)"=w246, "Current Limit (0.0 Amps)"=w242, "VISA resource name"=w247) -> ("error out"=w241:errorcluster)  [unwired: 7 in, 1 out]
        n87 = call-poly "Read.vi"("error in (no error)"=w241, "VISA resource name"=w240) -> ("error out"=w239:errorcluster, "Measurement"=w235:dbl)  [unwired: 7 in, 1 out]
        n88 = call-poly "Read.vi"("error in (no error)"=w239, "VISA resource name"=w238) -> ("error out"=w234:errorcluster, "Measurement"=w233:dbl)  [unwired: 7 in, 1 out]
        n89 = call <vilib>:"Add State(s) to Queue__jki_lib_state_machine.vi"("State(s) in (\"\")"=w249) -> ("States Out"=w248:string)  [unwired: 14 in]
        n90 = Bundle By Name(cluster=w236, "output_results.Vout 2 Measured(V)"=w235, "output_results.Vin 2 Measured (V)"=w233) -> (w237:T4)
      }
      frame "Test: Disable Supply and Load" {
        w255 = FALSE ("Output Enabled (F: Off)")
        n91 = Unbundle By Name(w258) -> ("instrument_resources.Vin_supply"=w256:refnum<visa-resource-name>, "instrument_resources.Vdd_supply"=w257:refnum<visa-resource-name>, "instrument_resources.Eload"=w250:refnum<visa-resource-name>)
        n92 = call "Close.vi"("error in (no error)"=w252, "VISA resource name"=w250) -> ("error out"=w251:errorcluster)  [unwired: 9 in]
        n93 = call "Configure Output Enabled.vi"("error in (no error)"=w251, "Output Enabled (F: Off)"=w255, "VISA resource name"=w257) -> ("error out"=w254:errorcluster)  [unwired: 7 in, 1 out]
        n94 = call "Configure Output Enabled.vi"("error in (no error)"=w254, "Output Enabled (F: Off)"=w255, "VISA resource name"=w256) -> ("error out"=w253:errorcluster)  [unwired: 7 in, 1 out]
        n95 = call <vilib>:"Add State(s) to Queue__jki_lib_state_machine.vi"("State(s) in (\"\")"=w260) -> ("States Out"=w259:string)  [unwired: 14 in]
      }
      frame "Test: Calculate Line Regulation" {
        n96 = Unbundle By Name(w272) -> ("output_results.Vin 1 Measured (V)"=w262:dbl, "output_results.Vin 2 Measured (V)"=w263:dbl, "output_results.Vout 1 Measured(V)"=w264:dbl, "output_results.Vout 2 Measured(V)"=w265:dbl)  [unwired: 1 out]
        n97 = Subtract(x=w265, y=w264) -> (x-y=w266:dbl)
        n98 = Subtract(x=w263, y=w262) -> (x-y=w270:dbl)
        n99 = Absolute Value(x=w266) -> (abs(x)=w267:dbl)
        n100 = Divide(x=w267, y=w264) -> (x/y=w271:dbl)
        n101 = Divide(x=w271, y=w270) -> (x/y=w269:dbl)
        n102 = Multiply(x=w269, y=1000000.0) -> (x*y=w261:dbl)
        n103 = Bundle By Name(cluster=w272, "output_results.Line Regulation ppm/v"=w261) -> (w273:T4)
        n104 = call <vilib>:"Add State(s) to Queue__jki_lib_state_machine.vi"("State(s) in (\"\")"=w276) -> ("States Out"=w275:string)  [unwired: 14 in]
      }
      frame "Test: Update Results to UI" {
        n105 = Unbundle By Name(w278) -> ("output_results"=→"Output Results":T2)
        n106 = call <vilib>:"Add State(s) to Queue__jki_lib_state_machine.vi"("State(s) in (\"\")"=w281) -> ("States Out"=w280:string)  [unwired: 14 in]
      }
    }
  }
